vi "0025ConfusingSwitches.vi"() -> ()   [LabVIEW 2010]
panel:
  out "The Light":bool
  in  "C":bool
  in  "B":bool
  in  "A":bool
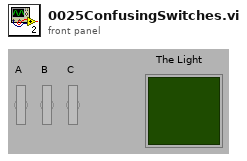
[diagram p1: front panel]
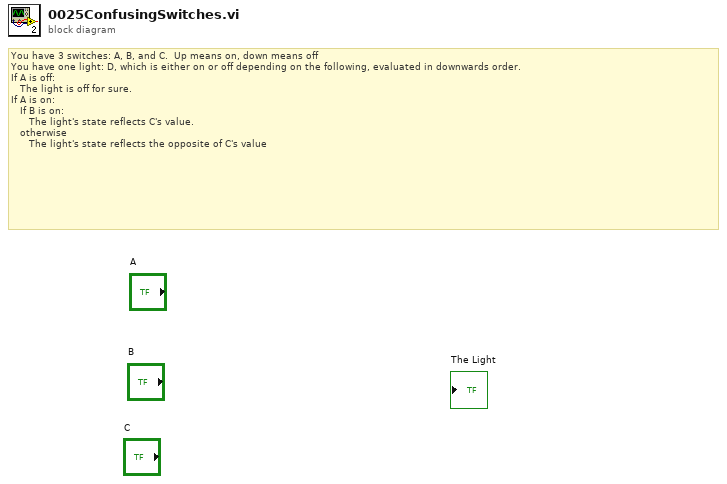
[diagram p0: block diagram]
diagram:
  # "You have 3 switches: A, B, and C.  Up means on, down means off\nYou have one light: D, which is either on or off depending on the following, evaluated in downwards order.\nIf A is off: \n   The light is off for sure.\nIf A is on:\n   If B is on:\n      The light's state reflects C's value.\n   otherwise\n      The light's state reflects the opposite of C's value"
